vi "Available parts Display.vi"(11 "error in":errorcluster) -> (6 "Part Number Out":string, 10 "Cancel?":bool, 14 "Part Number":string, 15 "error out":errorcluster)   [LabVIEW 2021]
panel:
  out "appended path":path
  in  "Vertical Cancel Button":bool
  in  "Vertical Open Button":bool
  in  "Select Model":i32(listbox)=10
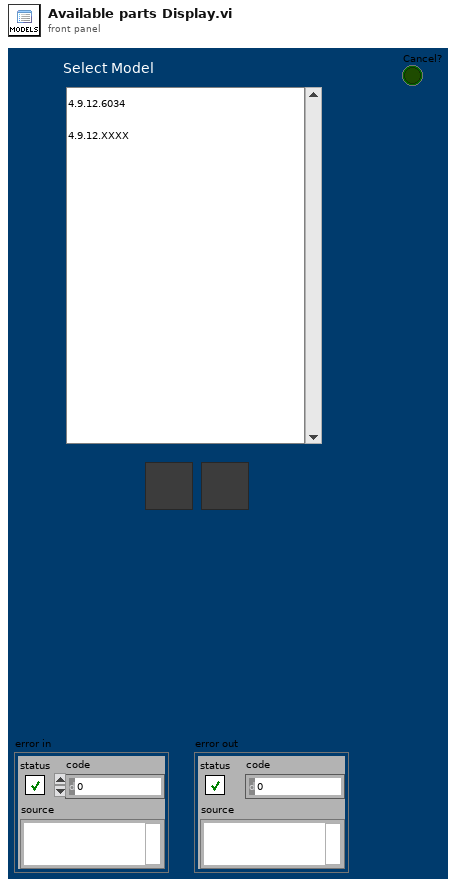
[diagram p1: front panel]
types:
  T1 = enum8{"Enabled", "Disabled", "Disabled and Grayed Out"}
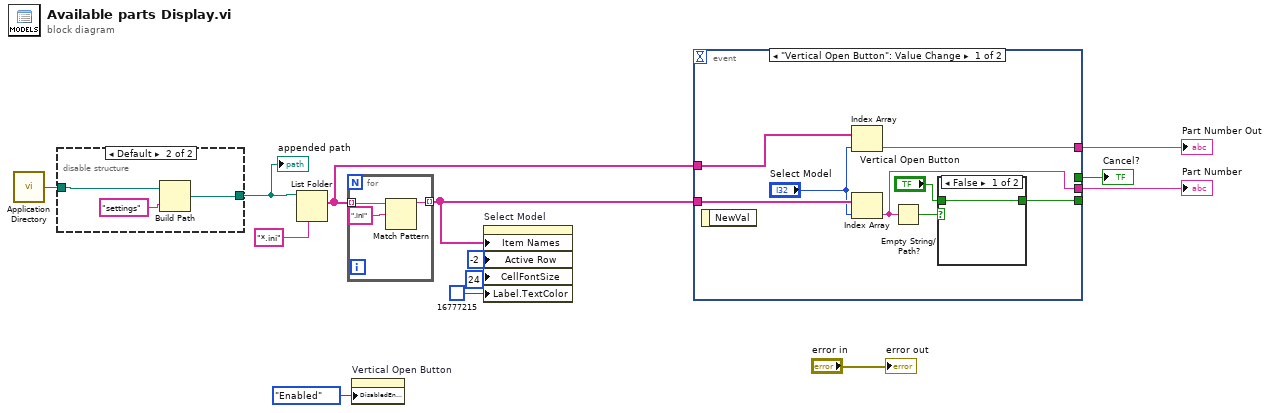
[diagram p0: block diagram]
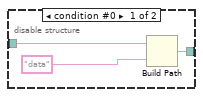
[diagram p2: hidden frame]
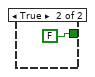
[diagram p3: hidden frame]
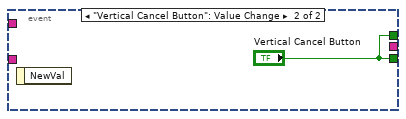
[diagram p4: hidden frame]
diagram:
  n1 = call <vilib>:"Application Directory.vi"() -> ("Application Directory"=w2:path)
  n2 = disable-structure shown="Default" {
    disable-tunnel: [w14 w17] -> w1
    disable-tunnel: w2 -> [w15 w18]
    frame condition #0 {
      n3 = Build Path(base path=w15, name or relative path="data") -> (appended path=w14:path)
    }
    frame condition #1 (active) {
      n4 = Build Path(base path=w18, name or relative path="settings") -> (appended path=w17:path)
    }
  }
  "appended path" <- w1
  n5 = List Folder(path=w1, pattern="*.ini") -> (filenames=w7:string[])  [unwired: 2 in, 3 out]
  n6 = for {
    tunnel: w7 -> [w21] mode=indexing
    tunnel: [w20] -> w12 mode=indexing
    n7 = Match Pattern(string=w21, regular expression=".ini") -> (before substring=w20:string)  [unwired: 1 in, 3 out]
  }
  n8 = property on="Vertical Open Button" class="Bool"("DisabledEnum"=T1."Enabled" ("Disabled")) -> ()  [unwired: 2 in, 2 out]
  n9 = property on="Select Model" class="LstBox (strict)"("Item Names"=w12, "Active Row"=-2 ("Active Row:Active Row Number"), "CellFontSize"=u32 24 ("Active Row:Cell Font:Size"), "Label.TextColor"=u32 16777215 ("Label.Text Colors:Text Color")) -> ()  [unwired: 2 in, 2 out]
  n10 = event shown="[0] \"Vertical Open Button\": Value Change" {
    selector: _ -> [_ _]
    dyn-events: _ -> [_ _]
    timeout: _ -> [_ _]
    tunnel: [_ "Vertical Cancel Button"] -> w4
    tunnel: [w29 "Vertical Cancel Button"] -> _
    tunnel: w12 -> [w27 _]
    tunnel: [w24 _] -> w9
    tunnel: w7 -> [w26 _]
    tunnel: [w23 _] -> w6
    event "Vertical Open Button": Value Change {
      n11 = event-data() -> ()  [unwired: 1 in, 1 out]
      n12 = Index Array(array=w26, index="Select Model") -> (element=w23:string)
      n13 = Index Array(array=w27, index="Select Model") -> (element=w24:string)
      n14 = Empty String/Path?(string/path=w24) -> (empty?=w30:bool)
      n15 = case shown="False" w30 {
        tunnel: [w31 FALSE ("Vertical Cancel Button")] -> w29
        tunnel: "Vertical Open Button" -> [w31 _]
        frame False {
        }
        frame True {
        }
      }
    }
    event "Vertical Cancel Button": Value Change {
      n16 = event-data() -> ()  [unwired: 1 in, 1 out]
    }
  }
  "Part Number" <- w9
  "Part Number Out" <- w6
  "Cancel?" <- w4
  "error out" <- "error in"
